vi "top_FreeMode.vi"(4 "Mode":enum16{"keypad", "button"}(ring), 5 "Cluster":T3, 6 "Volume":dbl=70.0) -> (1 "element":T2(ring), 2 "Boolean":bool=TRUE)   [LabVIEW 2014]
uses:
  <vilib>/sound2/lvsound2.llb/Sound Data Format.ctl
  <vilib>/sound2/lvsound2.llb/Sound Output Set Volume (Single).vi
  <vilib>/Utility/inputDevices.llb/keyboardAcquire.vi
  <vilib>/sound2/lvsound2.llb/Sound Output Write (DBL Single).vi
  <vilib>/Utility/inputDevices.llb/closeKeyboard.vi
  <vilib>/measure/NI_MABase.lvlib
panel:
  out "String":string
  in  "Song":T1(ring)
  in  "stop":bool
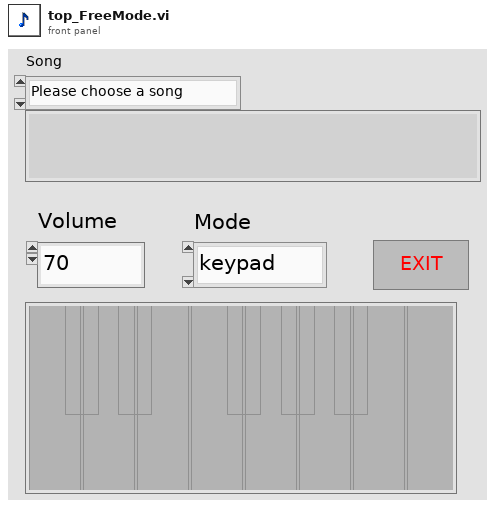
[diagram p1: front panel]
types:
  T1 = enum16{"Please choose a song", "two tiger", "little star"}
  T2 = enum16{"0", "1", "2", "3", "4", "5", "6", "7", "8", "9", "A", "B", "C", "D", "E", "F", "G", "H", "I", "J", "K", "L", "M", "N", "O", "P", "Q", "R", "S", "T", "U", "V", "W", "X", "Y", "Z", "F1", "F2", "F3", "F4", "F5", "F6", "F7", "F8", "F9", "F10", "F11", "F12", "F13", "F14", "F15", "ADD", "BACK", "BACKSLASH", "CAPITAL", "COMMA", "DECIMAL", "DELETE", "DIVIDE", "DOWN", "END", "EQUALS", "ESCAPE", "GRAVE (`)", "HOME", "INSERT", "LBRACKET", "LCONTROL", "LEFT", "L ALT", "LSHIFT", "LWIN", "MINUS", "MULTIPLY", "NEXT", "NUMLOCK", "NUMPAD_0", "NUMPAD_1", "NUMPAD_2", "NUMPAD_3", "NUMPAD_4", "NUMPAD_5", "NUMPAD_6", "NUMPAD_7", "NUMPAD_8", "NUMPAD_9", "PAUSE", "PERIOD", "PRIOR (PG UP)", "RBRACKET", "RCONTROL", "RETURN", "RIGHT", "R ALT", "RSHIFT", "RWIN", "SCROLL", "SEMICOLON", "SLASH", "SPACE", "SUBTRACT", "TAB", "UP", "ENTER (num pad)", "' (quote)"}
  T3 = cluster{"c 2":bool, "c 3":bool, "c 4":bool, "c 5":bool, "c 6":bool, "c 7":bool, "c 8":bool, "c 9":bool, "c":bool, "c 10":bool, "c 11":bool, "c 12":bool, "c 13":bool}
  T4 = typedef "Sound Data Format.ctl" = cluster{"sample rate (S/s)":dbl, "number of channels":i32, "bits per sample":i32}
  T5 = typedef "Sound Output Task ID.ctl" = u32
  T6 = cluster{"sample rate (S/s)":dbl, "number of samples/ch":i32}
  T7 = enum16{"0", "1", "2", "3", "4", "5", "6", "7", "8", "9", "A", "B", "C", "D", "E", "F", "G", "H", "I", "J", "K", "L", "M", "N", "O", "P", "Q", "R", "S", "T", "U", "V", "W", "X", "Y", "Z", "F1", "F2", "F3", "F4", "F5", "F6", "F7", "F8", "F9", "F10", "F11", "F12", "F13", "F14", "F15", "ADD", "BACK", "BACKSLASH", "CAPITAL", "COMMA", "DECIMAL", "DELETE", "DIVIDE", "DOWN", "END", "EQUALS", "ESCAPE", "GRAVE (`)", "HOME", "INSERT", "LBRACKET", "LCONTROL", "LEFT", "L ALT", "LSHIFT", "LWIN", "MINUS", "MULTIPLY", "NEXT", "NUMLOCK", "NUMPAD_0", "NUMPAD_1", "NUMPAD_2", "NUMPAD_3", "NUMPAD_4", "NUMPAD_5", "NUMPAD_6", "NUMPAD_7", "NUMPAD_8", "NUMPAD_9", "PAUSE", "PERIOD", "PRIOR (PG UP)", "RBRACKET", "RCONTROL", "RETURN", "RIGHT", "R ALT", "RSHIFT", "RWIN", "SCROLL", "SEMICOLON", "SLASH", "SPACE", "SUBTRACT", "TAB", "UP", "ENTER (num pad)", "' (quote)"}[]
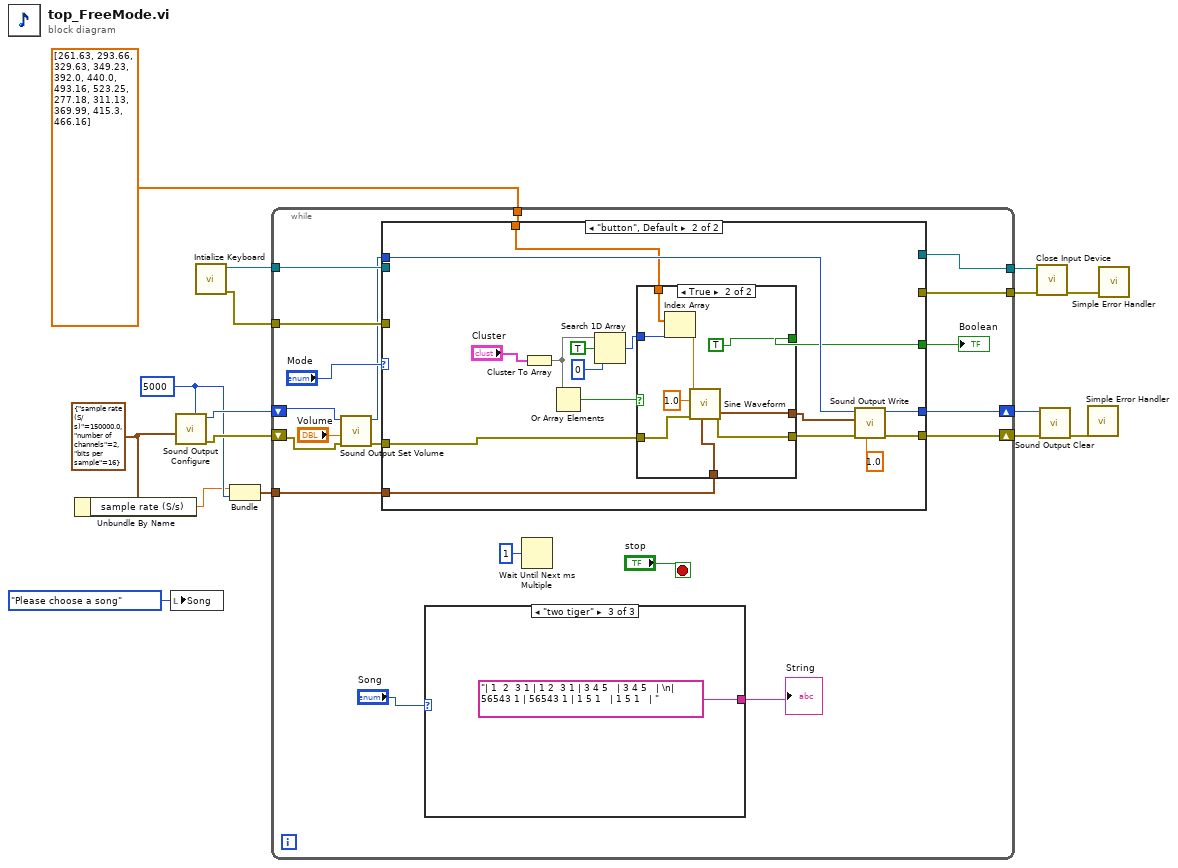
[diagram p0: block diagram]
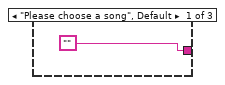
[diagram p2: hidden frame]
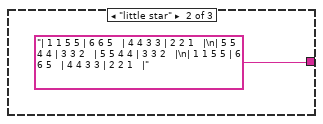
[diagram p3: hidden frame]
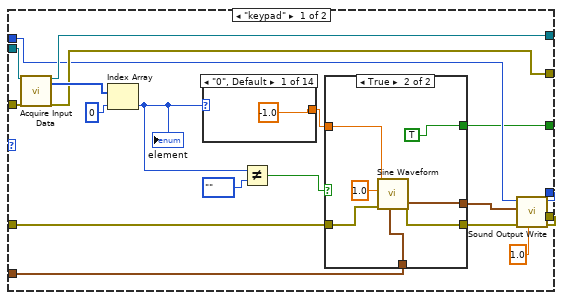
[diagram p4: hidden frame]
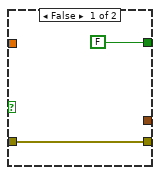
[diagram p5: hidden frame]
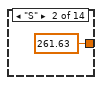
[diagram p6: hidden frame]
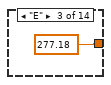
[diagram p7: hidden frame]
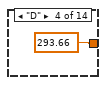
[diagram p8: hidden frame]
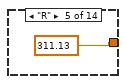
[diagram p9: hidden frame]
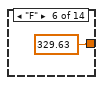
[diagram p10: hidden frame]
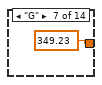
[diagram p11: hidden frame]
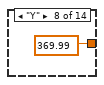
[diagram p12: hidden frame]
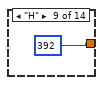
[diagram p13: hidden frame]
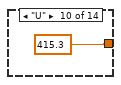
[diagram p14: hidden frame]
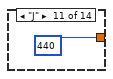
[diagram p15: hidden frame]
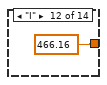
[diagram p16: hidden frame]
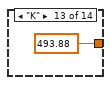
[diagram p17: hidden frame]
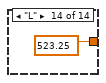
[diagram p18: hidden frame]
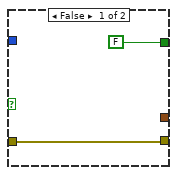
[diagram p19: hidden frame]
diagram:
  w13 = 5000 ("number of samples/ch")
  w14 = T4 {"sample rate (S/s)"=150000.0, "number of channels"=2, "bits per sample"=16} ("sound format")
  n1 = Unbundle By Name(w14) -> ("sample rate (S/s)"=w12:dbl)
  n2 = local write "Song"(T1."Please choose a song" ("Song")) -> ()
  n3 = call <vilib>:"Sound Output Configure.vi"("number of samples/ch"=w13, "sound format"=w14) -> ("error out"=w15:errorcluster, "task ID"=w16:T5)  [unwired: 8 in]
  n4 = call <vilib>:"Intialize Keyboard.vi"() -> ("error out"=w5:errorcluster, "device ID"=w4:refnum<k1>)  [unwired: 10 in]
  n5 = Bundle("sample rate (S/s)"=w12, "number of samples/ch"=w13) -> (w11:T6)  [unwired: 1 in]
  n6 = while {
    tunnel: w11 -> [w32]
    tunnel: dbl[] [261.63, 293.66, 329.63, 349.23, 392.0, 440.0, 493.16, 523.25, 277.18, 311.13, 369.99, 415.3, 466.16] -> [w28]
    shift-right: [w31] -> w10
    shift-left: w16 -> [w34]
    shift-right: [w30] -> w9
    shift-left: w15 -> [w29]
    tunnel: w5 -> [w24]
    tunnel: w4 -> [w23]
    tunnel: [w22] -> w3
    tunnel: [w21] -> w2
    stop <- "stop" stop-if-true
    n7 = call-poly <vilib>:"Sound Output Set Volume.vi"("error in (no error)"=w29, "volume"="Volume", "task ID"=w34) -> ("error out"=w33:errorcluster, "task ID out"=w20:T5)  [unwired: 7 in]
    n8 = case shown="\"button\", Default" "Mode" {
      tunnel: w33 -> [w44 w96]
      tunnel: w32 -> [w43 w93]
      tunnel: w20 -> [w42 w92]
      tunnel: [w41 w91] -> w31
      tunnel: [w40 w90] -> w30
      tunnel: w28 -> [_ w89]
      tunnel: w24 -> [w48 _]
      tunnel: w23 -> [w47 _]
      tunnel: [w46 _] -> w22
      tunnel: [w45 _] -> w21
      tunnel: [w39 w81] -> w19
      frame "keypad" {
        n9 = call-poly <vilib>:"Acquire Input Data.vi"("device ID"=w47, "error in (no error)"=w48) -> ("device ID"=w46:refnum<k1>, "keys pressed"=w53:T7, "error out"=w45:errorcluster)  [unwired: 15 in]
        n10 = Index Array(array=w53, index=0) -> (element=w57:T2)
        "element" <- w57
        n11 = case shown="\"0\", Default" w57 {
          tunnel: [-1.0 261.63 277.18 293.66 311.13 329.63 349.23 369.99 392 415.3 440 466.16 493.88 523.25] -> w52
          frame "0", Default {
          }
          frame "S" {
          }
          frame "E" {
          }
          frame "D" {
          }
          frame "R" {
          }
          frame "F" {
          }
          frame "G" {
          }
          frame "Y" {
          }
          frame "H" {
          }
          frame "U" {
          }
          frame "J" {
          }
          frame "I" {
          }
          frame "K" {
          }
          frame "L" {
          }
        }
        n12 = Not Equal?(x=w57, y=enum16{""}."") -> (x != y?=w56:bool)
        n13 = case shown="True" w56 {
          tunnel: w44 -> [w59 w65]
          tunnel: [_ w64] -> w49
          tunnel: [w59 w63] -> w50
          tunnel: w43 -> [_ w62]
          tunnel: w52 -> [_ w61]
          tunnel: [FALSE TRUE] -> w39
          frame False {
          }
          frame True {
            n14 = call <vilib>:"Sine Waveform.vi"("sampling info"=w62, "error in (no error)"=w65, "amplitude"=1.0, "frequency"=w61) -> ("error out"=w63:errorcluster, "signal out"=w64:waveform(dbl))  [unwired: 6 in]
          }
        }
        n15 = call-poly <vilib>:"Sound Output Write.vi"("timeout (sec)"=1.0, "error in (no error)"=w50, "data"=w49, "task ID"=w42) -> ("error out"=w40:errorcluster, "task ID out"=w41:T5)  [unwired: 6 in]
      }
      frame "button", Default {
        n16 = Cluster To Array(cluster="Cluster") -> (array=w84:bool[])
        n17 = Or Array Elements(Boolean array=w84) -> (logical OR=w83:bool)
        n18 = Search 1D Array(1D array=w84, element=TRUE, start index (0)=0) -> (index of element=w82:i32)
        n19 = case shown="True" w83 {
          tunnel: w96 -> [w98 w106]
          tunnel: [_ w105] -> w95
          tunnel: [w98 w104] -> w94
          tunnel: w93 -> [_ w103]
          tunnel: w89 -> [_ w102]
          tunnel: w82 -> [_ w101]
          tunnel: [FALSE TRUE] -> w81
          frame False {
          }
          frame True {
            n20 = Index Array(array=w102, index=w101) -> (element=w100:dbl)
            n21 = call <vilib>:"Sine Waveform.vi"("sampling info"=w103, "error in (no error)"=w106, "amplitude"=1.0, "frequency"=w100) -> ("error out"=w104:errorcluster, "signal out"=w105:waveform(dbl))  [unwired: 6 in]
          }
        }
        n22 = call-poly <vilib>:"Sound Output Write.vi"("timeout (sec)"=1.0, "error in (no error)"=w94, "data"=w95, "task ID"=w92) -> ("error out"=w90:errorcluster, "task ID out"=w91:T5)  [unwired: 6 in]
      }
    }
    "Boolean" <- w19
    n23 = case shown="\"two tiger\"" "Song" {
      tunnel: ["" "| 1 1 5 5 | 6 6 5   | 4 4 3 3 | 2 2 1   |\n| 5 5 4 4 | 3 3 2   | 5 5 4 4 | 3 3 2   |\n| 1 1 5 5 | 6 6 5   | 4 4 3 3 | 2 2 1   |" "| 1  2  3 1 | 1 2  3 1 | 3 4 5   | 3 4 5   | \n| 56543 1 | 56543 1 | 1 5 1   | 1 5 1   | "] -> w17
      frame "Please choose a song", Default {
      }
      frame "little star" {
      }
      frame "two tiger" {
      }
    }
    "String" <- w17
    n24 = Wait Until Next ms Multiple(millisecond multiple=u32 1) -> ()  [unwired: 1 out]
  }
  n25 = call-poly <vilib>:"Close Input Device.vi"("error in (no error)"=w2, "device ID"=w3) -> ("error out"=w6:errorcluster)  [unwired: 8 in]
  n26 = call <vilib>:"Sound Output Clear.vi"("error in (no error)"=w9, "task ID"=w10) -> ("error out"=w8:errorcluster)  [unwired: 9 in]
  n27 = call <vilib>:"Simple Error Handler.vi"("error in (no error)"=w8) -> ()  [unwired: 4 in, 5 out]
  n28 = call <vilib>:"Simple Error Handler.vi"("error in (no error)"=w6) -> ()  [unwired: 4 in, 5 out]
